vi "Query Voltage.vi"(8 "error in (no error)":errorcluster, 11 "Manual PSU in":refnum<class "Manual PSU.lvclass">) -> (0 "error out":errorcluster, 2 "Voltage":dbl, 3 "Manual PSU out":refnum<class "Manual PSU.lvclass">)   [LabVIEW 2020, in "Manual PSU.lvclass"]
uses:
  Manual PSU.lvclass
  C:/Sandbox/RF Bench/Source Code/WiSpry Test Framework/Instruments/Power Supply/Power Supply.lvclass
  Power Supply.lvclass/Power Supply.ctl
  Power Supply.lvclass
panel:
  out "OK":bool
  in  "Enable":bool=TRUE
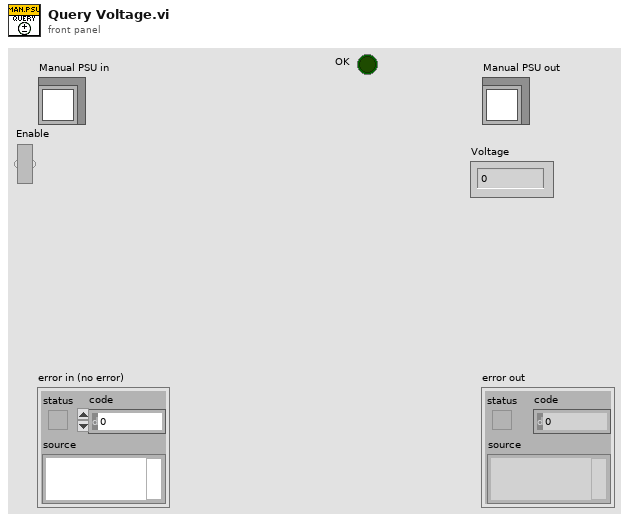
[diagram p1: front panel]
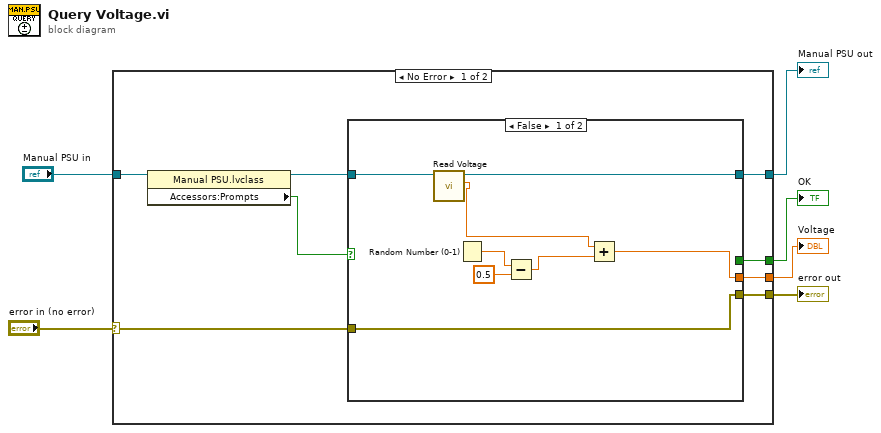
[diagram p0: block diagram]
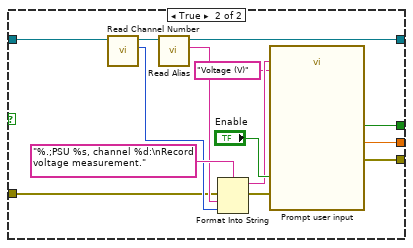
[diagram p2: hidden frame]
diagram:
  n1 = case shown="No Error" "error in (no error)" {
    selector: "error in (no error)" -> [w10 w37]
    tunnel: "Manual PSU in" -> [w9 w38]
    tunnel: [w14 w38] -> w5
    tunnel: [w13 _] -> w4
    tunnel: [w12 w37] -> w3
    tunnel: [w11 _] -> w2
    frame No Error {
      n2 = property class="Manual PSU.lvclass"(reference=w9) -> (reference out=w8:refnum<class "Manual PSU.lvclass">, "Accessors:Prompts"=w7:bool)  [unwired: 1 in, 1 out]
      n3 = case shown="False" w7 {
        tunnel: w8 -> [w21 w35]
        tunnel: [w20 w34] -> w14
        tunnel: [w15 w33] -> w13
        tunnel: [w22 w32] -> w12
        tunnel: [_ w30] -> w11
        tunnel: w10 -> [w22 w24]
        frame False {
          n4 = call "Read Voltage.vi"("Power Supply in"=w21) -> ("Voltage"=w16:dbl, "Power Supply out"=w20:refnum<class "Manual PSU.lvclass">)  [unwired: 9 in]
          n5 = Random Number (0-1)() -> (number: 0 to 1=w19:dbl)
          n6 = Subtract(x=w19, y=0.5) -> (x-y=w17:dbl)
          n7 = Add(x=w16, y=w17) -> (x+y=w15:dbl)
        }
        frame True {
          n8 = call "Read Channel Number.vi"("Power Supply in"=w35) -> ("Channel Number"=w27:u8, "Power Supply out"=w36:refnum<class "Manual PSU.lvclass">)  [unwired: 9 in]
          n9 = call-dynamic "Read Alias.vi"("Power Supply in"=w36) -> ("Alias"=w28:string, "Power Supply out"=w34:refnum<class "Manual PSU.lvclass">)  [unwired: 9 in]
          n10 = Format Into String(format string="%.;PSU %s, channel %d:\nRecord voltage measurement.", error in=w24, w28, w27) -> (resulting string=w25:string, error out=w26:errorcluster)  [unwired: 1 in]
          n11 = call "Prompt user input.vi"("Enable"="Enable", "String"=w25, "Parameter Caption"="Voltage (V)", "error in (no error)"=w26) -> ("output"=w33:dbl, "OK"=w30:bool, "error out"=w32:errorcluster)  [unwired: 13 in]
        }
      }
    }
    frame Error {
    }
  }
  "error out" <- w3
  "Manual PSU out" <- w5
  "Voltage" <- w4
  "OK" <- w2
